vi "ini Open File.vi"(0 "ini File":path, 5 "Error In":errorcluster) -> (14 "ini Refnum":T1, 19 "Error Out":errorcluster)   [LabVIEW 2019, in "Application.lvclass"]
uses:
  Application.lvclass
  <vilib>/Utility/config.llb/Config Data RefNum.ctl
  <vilib>/Utility/config.llb/NI_LVConfig.lvlib
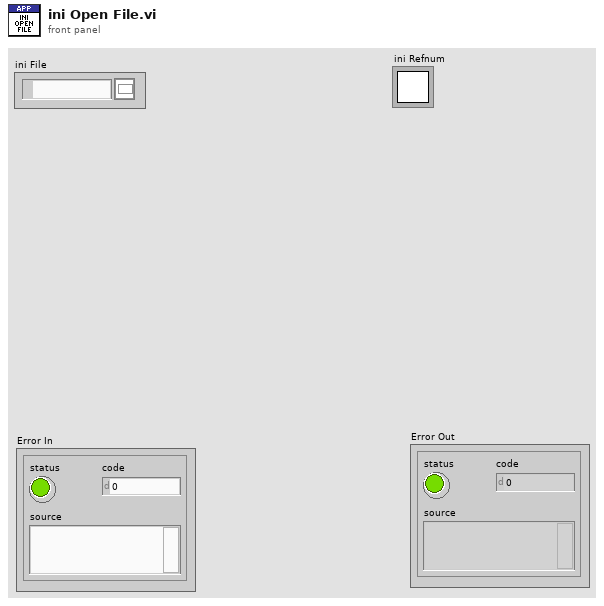
[diagram p1: front panel]
types:
  T1 = typedef "NI_LVConfig.lvlib/Config Data RefNum.ctl" = refnum<k1>
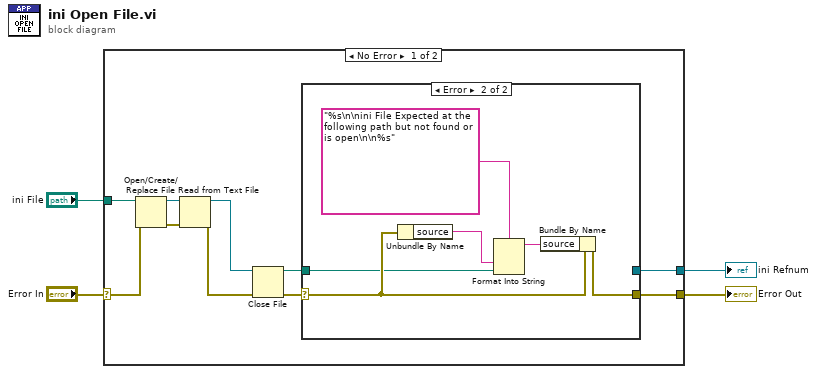
[diagram p0: block diagram]
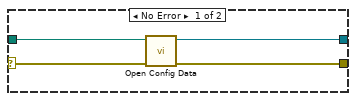
[diagram p2: hidden frame]
diagram:
  n1 = case shown="No Error" "Error In" {
    selector: "Error In" -> [w14 w25]
    tunnel: "ini File" -> [w13 _]
    tunnel: [w12 _] -> w2
    tunnel: [w5 w25] -> w1
    frame No Error {
      n2 = Open/Create/Replace File(file path (use dialog)=w13, error in=w14) -> (refnum out=w11:refnum<file>, error out=w10:errorcluster)  [unwired: 4 in, 1 out]
      n3 = Read from Text File(file (use dialog)=w11, error in=w10) -> (refnum out=w8:refnum<file>, error out=w9:errorcluster)  [unwired: 2 in, 2 out]
      n4 = Close File(refnum=w8, error in=w9) -> (path=w6:path, error out=w7:errorcluster)
      n5 = case shown="Error" w7 {
        selector: w7 -> [w17 w24]
        tunnel: w6 -> [w18 w22]
        tunnel: [w16 _] -> w12
        tunnel: [w15 w19] -> w5
        frame No Error {
          n6 = call <vilib>:"Open Config Data.vi"("error in (no error)"=w17, "configuration file path"=w18) -> ("error out"=w15:errorcluster, "refnum"=w16:T1)  [unwired: 7 in, 1 out]
        }
        frame Error {
          n7 = Unbundle By Name(w24) -> ("source"=w23:string)
          n8 = Format Into String(format string="%s\n\nini File Expected at the following path but not found or is open\n\n%s", w23, w22) -> (resulting string=w20:string)  [unwired: 2 in, 1 out]
          n9 = Bundle By Name(cluster=w24, "source"=w20) -> (w19:errorcluster)
        }
      }
    }
    frame Error {
    }
  }
  "Error Out" <- w1
  "ini Refnum" <- w2
